vi "ingest.job_rid.vi"(8 "error in":errorcluster, 11 "IngestJob in":refnum<class "IngestJob.lvclass">) -> (0 "error out":errorcluster, 3 "IngestJob out":refnum<class "IngestJob.lvclass">)   [LabVIEW 2020, in "IngestJob.lvclass"]
doc: "Returns the identifier of an ingest job."
uses:
  IngestJob.lvclass
  IngestJob.lvclass/IngestJob.ctl
  client.lvlib
panel:
  out "out_needed out":u32
  out "job rid":string
  in  "buf":string
  in  "cap":u32
  in  "out_needed":u32
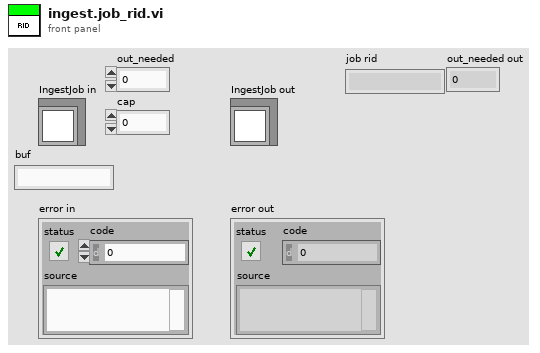
[diagram p1: front panel]
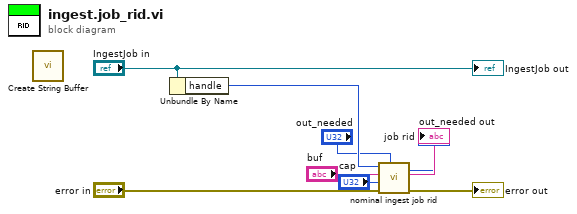
[diagram p0: block diagram]
diagram:
  n1 = call "Create String Buffer.vi"() -> ()  [unwired: 9 in, 3 out]
  n2 = Unbundle By Name("IngestJob in") -> ("handle"=w7:i32)
  n3 = call "nominal ingest job rid.vi"("out_needed"="out_needed", "error in (no error)"="error in", "cap"="cap", "buf"="buf", "job"=w7) -> ("error out"=→"error out":errorcluster, "buf out"=→"job rid":string, "out_needed out"=→"out_needed out":u32)  [unwired: 3 in, 1 out]
  "IngestJob out" <- "IngestJob in"
